vi "test_rd_xctl.vi"() -> ()   [LabVIEW 2012]
uses:
  Ringdown.xctl
panel:
  in  "Boolean":bool
  out "Ringdown":i16[][][](xcontrol)
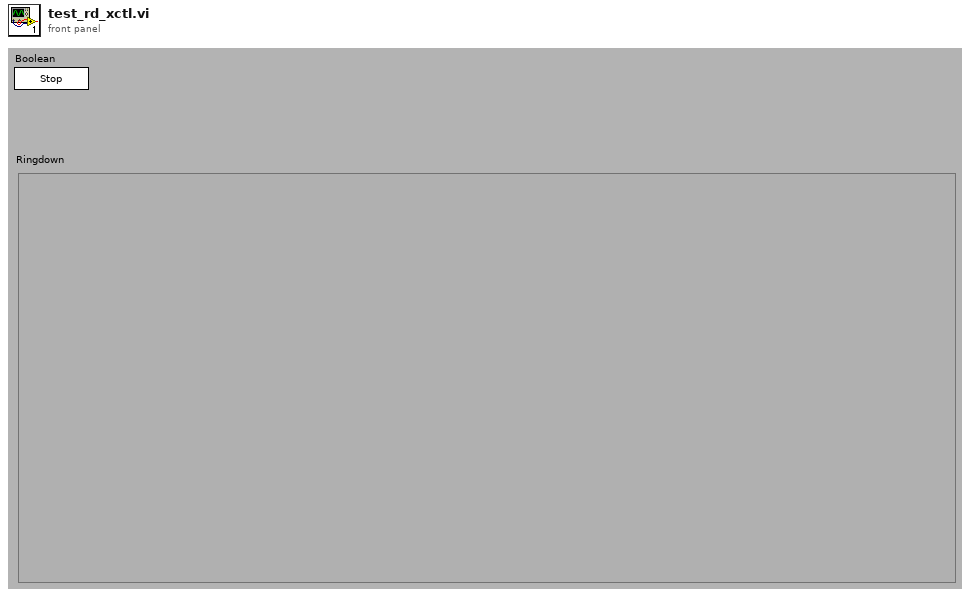
[diagram p1: front panel]
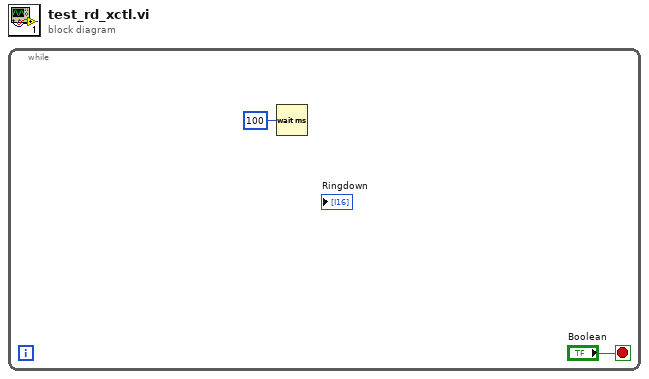
[diagram p0: block diagram]
diagram:
  n1 = while {
    stop <- "Boolean" stop-if-true
    n2 = Wait (ms)(milliseconds to wait=u32 100) -> ()  [unwired: 1 out]
  }
